vi "Set Indicator LEDs.vi"(8 "error in (no error)":errorcluster, 10 "LED Index":i32, 11 "Color":u32(colorbox)) -> (0 "error out":errorcluster)   [LabVIEW 2019]
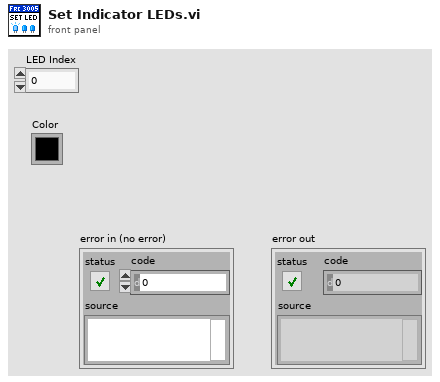
[diagram p1: front panel]
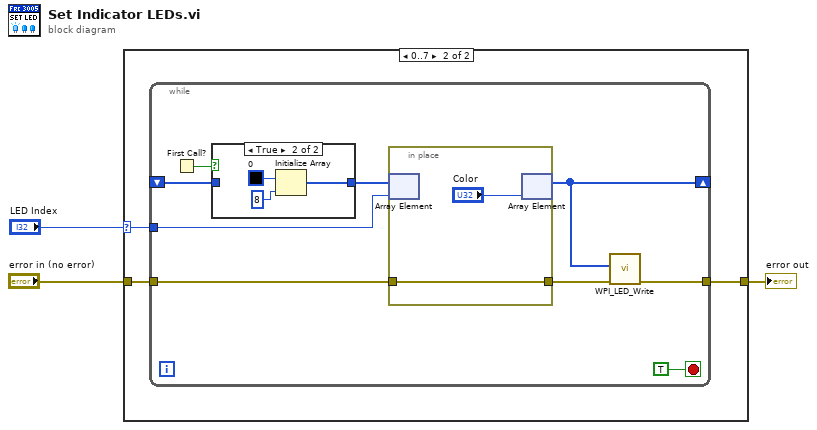
[diagram p0: block diagram]
diagram:
  n1 = case shown="0..7" "LED Index" {
    selector: "LED Index" -> [_ w5]
    tunnel: "error in (no error)" -> [w4 w7]
    tunnel: [w4 w6] -> w2
    frame Default {
    }
    frame 0..7 {
      n2 = while {
        shift-right: [w11] -> _
        shift-left: _ -> [w9]
        tunnel: w5 -> [w15]
        tunnel: w7 -> [w14]
        tunnel: [w12] -> w6
        stop <- TRUE stop-if-true
        n3 = First Call?() -> (First Call?: T/F=w10:bool)
        n4 = case shown="True" w10 {
          tunnel: [w17 w18] -> w8
          tunnel: w9 -> [w17 _]
          frame False {
          }
          frame True {
            n5 = Initialize Array(u32 0 ("Color"), 8 ("dimension size")) -> (w18:u32[])
          }
        }
        n6 = in-place {
          in-place-border: w14 -> [w22]
          in-place-border: [w22] -> w13
          n7 = in-place-array #1(w8, w15) -> ()  [unwired: 1 out]
          n8 = in-place-array #1("Color") -> (w11:u32[])  [unwired: 1 out]
        }
        n9 = call <vilib>:"WPI_LED_Write.vi"("error in"=w13, "Color Array"=w11) -> ("error out"=w12:errorcluster)  [unwired: 9 in]
      }
    }
  }
  "error out" <- w2
